vi "Configuration file.vi"(8 "error in (no error)":errorcluster caption="错误输入（无错误）", 11 "类型":enum16{"读取", "写入"}(ring)) -> (0 "error out":errorcluster caption="错误输出")   [LabVIEW 2016, in "EXO2-Sonde.lvlib"]
uses:
  EXO2-Sonde.lvlib
  Var/Holding Var.vi
  <vilib>/Utility/config.llb/NI_LVConfig.lvlib
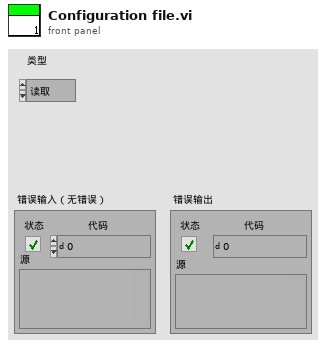
[diagram p1: front panel]
types:
  T1 = typedef "NI_LVConfig.lvlib/Config Data RefNum.ctl" = refnum<k1>
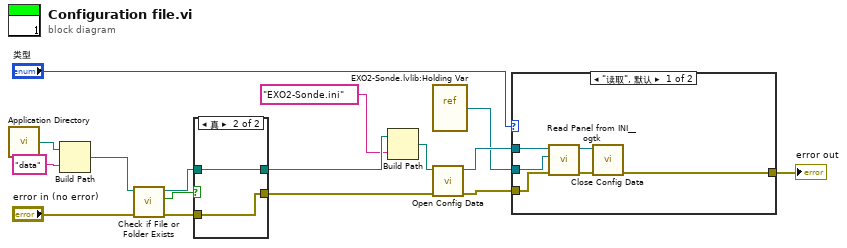
[diagram p0: block diagram]
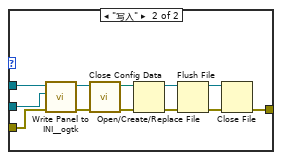
[diagram p2: hidden frame]
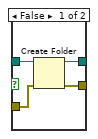
[diagram p3: hidden frame]
diagram:
  n1 = call <vilib>:"Application Directory.vi"() -> ("Application Directory"=w13:path)
  n2 = Build Path(base path=w13, name or relative path="data" ("名称或相对路径")) -> (appended path=w11:path)
  n3 = call <vilib>:"Check if File or Folder Exists.vi"("error in (no error)"="error in (no error)", "path"=w11) -> ("error out"=w8:errorcluster, "file or folder exists?"=w10:bool, "dup path"=w9:path)  [unwired: 7 in]
  n4 = case shown="真" w10 {
    tunnel: w9 -> [w20 w22]
    tunnel: w8 -> [w19 w21]
    tunnel: [w18 w22] -> w5
    tunnel: [w17 w21] -> w6
    frame False {
      n5 = Create Folder(path (use dialog)=w20, error in=w19) -> (created path=w18:path, error out=w17:errorcluster)  [unwired: 1 in, 1 out]
    }
    frame True {
    }
  }
  n6 = Build Path(base path=w5, name or relative path="EXO2-Sonde.ini" ("名称或相对路径")) -> (appended path=w3:path)
  n7 = vi-ref "EXO2-Sonde.lvlib:Holding Var.vi"() -> (w2:refnum<vi>)
  n8 = call <vilib>:"Open Config Data.vi"("error in (no error)"=w6, "configuration file path"=w3) -> ("error out"=w16:errorcluster, "refnum"=w15:T1)  [unwired: 7 in, 1 out]
  n9 = case shown="\"读取\", 默认" "类型" {
    tunnel: w16 -> [w25 w40]
    tunnel: w15 -> [w26 w39]
    tunnel: [w24 w30] -> w14
    tunnel: w2 -> [w23 w29]
    frame "读取", Default {
      n10 = call <userlib>:"Read Panel from INI__ogtk.vi"("error in (no error)"=w25, "VI ref"=w23, "refnum"=w26) -> ("error out"=w28:errorcluster, "refnum out"=w27:T1)  [unwired: 7 in]
      n11 = call <vilib>:"Close Config Data.vi"("error in (no error)"=w28, "refnum"=w27) -> ("error out"=w24:errorcluster)  [unwired: 8 in, 1 out]
    }
    frame "写入" {
      n12 = call <userlib>:"Write Panel to INI__ogtk.vi"("error in (no error)"=w40, "VI ref"=w29, "refnum"=w39) -> ("error out"=w38:errorcluster, "refnum out"=w37:T1)  [unwired: 7 in]
      n13 = call <vilib>:"Close Config Data.vi"("error in (no error)"=w38, "refnum"=w37) -> ("error out"=w31:errorcluster, "file path"=w32:path)  [unwired: 8 in]
      n14 = Open/Create/Replace File(file path (use dialog)=w32, error in=w31) -> (refnum out=w36:refnum<file>, error out=w35:errorcluster)  [unwired: 4 in, 1 out]
      n15 = Flush File(refnum=w36, error in=w35) -> (refnum out=w34:refnum<file>, error out=w33:errorcluster)
      n16 = Close File(refnum=w34, error in=w33) -> (error out=w30:errorcluster)  [unwired: 1 out]
    }
  }
  "error out" <- w14
